vi "2021 Advent puzzle 02.vi"() -> ()   [LabVIEW 2021]
panel:
  out "output 1":string
  out "64bit integer":i64
  out "index 2":i64
  out "index":i64
  out "x*y":i64
  out "y":i64
  out "x":i64
  # "1451208"
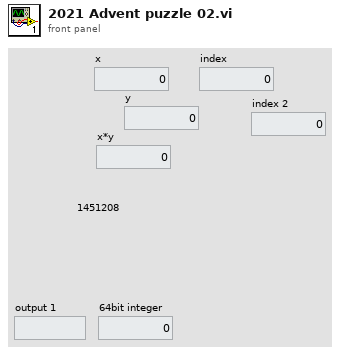
[diagram p1: front panel]
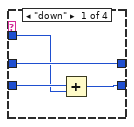
[diagram p2: hidden frame]
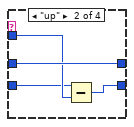
[diagram p3: hidden frame]
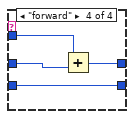
[diagram p4: hidden frame]
diagram:
  w5 = i64 0 ("index")
  (unwired) "forward 5\ndown 5\nforward 8\nup 3\ndown 8\nforward 2"
  # "find end position"
  n1 = Spreadsheet String To Array(delimiter (Tab)="\n", format string="", spreadsheet string="forward 9\ndown 3\ndown 8\nforward 2\nup 3\nforward 5\nup 8\ndown 2\ndown 5\nup 7\ndown 9\nforward 4\nup 5\ndown 9\nforward 2\nforward 2\nforward 8\ndown 6\nforward 2\nup 9\nup 5\ndown 2\nforward 5\ndown 8\nforward 3\nup 4\nforward 5\nforward 7\ndown 8\ndown 6\nup 7\ndown 3\nforward 4\nup 8\ndown 5\ndown 3\ndown 6\ndown 8\nforward 1\nforward 9\nforward 4\nup 7\ndown 4\nforward 7\nforward 3\nforward 9\ndown 1\ndown 3\nup 9\ndown 3\nforward 9\nup 6\nup 9\ndown 8\nup 3\ndown 1\nup 8\ndown 8\ndown 2\ndown 4\ndown 4\nup 3\ndown 6\ndown 1\ndown 3\nforward 1\nup 5\nforward 5\nforward 8\ndown 2\nforward 6\nforward 2\nup 7\nforward 6\ndown 8\nforward 6\nforward 5\nup 9\nforward 5\nup 5\nforward 9\ndown 2\ndown 4\ndown 3\ndown 8\nforward 9\nforward 6\nforward 2\nup 7\ndown 7\nup 3\nforward 4\nforward 5\ndown 7\nforward 5\nup 9\nforward 6\nforward 6\nforward 1\ndown 6\nforward 9\nup 2\ndown 7\ndown 8\ndown 6\nup 5\ndown 8\ndown 8\nforward 7\ndown 6\nup 5\ndown 9\ndown 3\nforward 2\ndown 4\nforward 8\ndown 5\nup 5\nforward 7\nup 2\nup 2\ndown 4\nforward 4\ndown 5\nup 8\ndown 2\nforward 4\ndown 9\nforward 8\ndown 5\ndown 6\ndown 7\nup 7\nup 5\nup 7\nforward 7\nforward 8\ndown 2\nforward 3\ndown 2\ndown 7\ndown 4\ndown 2\nforward 3\nforward 5\ndown 3\ndown 7\nup 7\ndown 7\nup 5\nforward 1\ndown 8\ndown 2\nup 4\nup 5\ndown 8\nforward 9\ndown 3\ndown 9\nforward 8\nforward 1\nforward 1\ndown 2\nup 9\ndown 2\nup 8\ndown 6\nup 8\nforward 7\ndown 5\nforward 7\ndown 8\nforward 8\ndown 7\nup 9\nup 2\nup 6\ndown 5\ndown 9\nforward 2\nup 3\ndown 4\nup 5\nup 4\ndown 9\nforward 7\nforward 7\ndown 3\nforward 4\nforward 9\nup 8\nforward 3\ndown 1\nforward 2\ndown 7\ndown 3\ndown 7\ndown 7\nforward 8\nforward 4\nforward 7\nup 1\ndown 4\nup 9\ndown 2\ndown 1\nforward 6\ndown 3\nforward 7\nforward 8\nup 9\nup 2\nup 2\nforward 7\nup 2\nup 5\nforward 5\ndown 3\nforward 8\nforward 1\nup 4\ndown 6\ndown 5\nforward 4\nup 9\nforward 8\nup 4\ndown 8\ndown 3\ndown 3\ndown 7\nforward 2\nforward 4\ndown 9\ndown 7\ndown 2\nup 3\nup 3\nforward 8\nforward 7\nforward 8\ndown 5\nup 5\nforward 3\nforward 6\nup 7\nup 1\nforward 2\nforward 5\ndown 5\nforward 8\ndown 2\ndown 4\nforward 2\ndown 7\ndown 3\ndown 5\nforward 9\ndown 7\ndown 8\nup 1\nup 2\ndown 8\nforward 7\nforward 8\ndown 8\nforward 5\nup 7\nforward 3\nup 2\ndown 7\nforward 1\ndown 2\nup 7\nup 4\ndown 2\nforward 1\nup 5\nforward 2\nup 2\nforward 3\nforward 9\nforward 2\nforward 8\nforward 2\nup 7\ndown 8\ndown 7\nforward 2\nforward 7\ndown 1\nforward 2\nup 1\nup 6\ndown 3\ndown 6\nforward 7\ndown 4\nforward 5\nforward 6\nup 3\nforward 3\ndown 6\nforward 8\nup 8\nforward 4\ndown 3\nforward 3\ndown 4\ndown 7\nforward 9\nforward 2\nup 2\nforward 8\ndown 6\nforward 6\ndown 9\ndown 9\nforward 8\ndown 1\nforward 9\ndown 1\ndown 6\ndown 8\ndown 5\ndown 5\nforward 3\nforward 3\ndown 2\ndown 5\nforward 9\ndown 2\ndown 8\ndown 3\nforward 9\nup 2\ndown 4\ndown 9\nforward 9\nforward 1\nforward 5\nup 9\ndown 1\ndown 6\nforward 6\nforward 5\nforward 8\ndown 2\nforward 8\ndown 4\ndown 2\ndown 6\ndown 6\nup 3\nup 8\nforward 1\ndown 1\nup 8\ndown 3\ndown 4\nup 9\nup 1\ndown 7\ndown 7\nup 1\nup 2\nforward 5\nup 8\nforward 2\ndown 3\nforward 1\nup 5\nforward 6\nforward 2\ndown 6\nup 2\nforward 2\nforward 1\ndown 3\nforward 4\nup 8\nforward 5\ndown 4\nforward 2\ndown 8\ndown 7\nup 7\ndown 8\nforward 1\ndown 4\nup 9\ndown 6\nup 6\nup 6\ndown 2\nforward 1\nforward 8\ndown 6\nup 3\ndown 7\nforward 9\nup 1\nup 4\nforward 7\ndown 7\nforward 1\ndown 6\ndown 4\ndown 7\ndown 8\ndown 8\nforward 4\ndown 6\ndown 6\ndown 5\nforward 6\nup 9\nup 3\ndown 4\nforward 8\ndown 7\nforward 6\nup 3\nforward 1\nforward 1\ndown 8\nforward 7\nforward 4\nforward 6\nup 1\nforward 7\nup 8\nforward 2\nforward 6\nforward 8\ndown 9\ndown 8\nup 9\nup 4\nup 2\nforward 2\nforward 8\nup 2\nforward 3\nforward 2\nup 2\nup 5\nup 8\nforward 4\nforward 8\nforward 3\nup 5\ndown 1\nforward 2\ndown 7\ndown 8\nforward 3\nup 1\nforward 5\nforward 7\nforward 9\nup 7\nforward 4\ndown 4\nup 2\nforward 4\nforward 5\nforward 3\nup 9\nforward 6\nforward 8\ndown 9\ndown 1\nforward 1\ndown 5\ndown 2\nforward 9\ndown 2\nup 9\ndown 1\nforward 5\nforward 8\nup 2\nforward 6\ndown 4\ndown 9\nforward 4\nforward 1\ndown 3\ndown 3\nup 5\nforward 5\ndown 6\nforward 3\ndown 2\nforward 8\ndown 7\ndown 2\ndown 1\nforward 2\nup 5\nforward 9\nforward 3\nforward 5\ndown 4\nup 7\nforward 6\ndown 3\nforward 1\nforward 7\nforward 1\nup 4\ndown 2\ndown 7\nup 9\nforward 9\ndown 8\ndown 1\nup 2\ndown 3\nforward 7\ndown 8\ndown 5\ndown 5\nup 8\nforward 1\ndown 5\nforward 8\nup 7\ndown 1\nforward 9\ndown 4\nforward 8\nforward 5\nforward 7\nforward 8\nforward 3\nup 9\nforward 3\ndown 7\ndown 5\nup 8\nforward 3\nup 6\nforward 8\nup 3\ndown 5\nforward 5\nforward 6\nforward 4\nforward 3\nforward 8\nup 9\nforward 2\ndown 6\ndown 4\ndown 5\nforward 7\ndown 2\nup 5\nforward 2\nforward 5\ndown 9\nforward 8\ndown 8\nforward 6\ndown 9\ndown 7\nup 9\nforward 3\nforward 3\nup 5\ndown 2\nforward 5\ndown 6\ndown 6\ndown 2\ndown 3\ndown 4\nforward 7\nup 1\ndown 7\nforward 7\nup 1\nforward 3\nup 6\ndown 7\ndown 5\nforward 9\nforward 2\ndown 5\nforward 9\ndown 5\nforward 9\nforward 1\ndown 4\nforward 9\ndown 5\nforward 8\ndown 6\ndown 4\ndown 5\nforward 9\ndown 1\nforward 6\nforward 9\ndown 1\ndown 1\nup 2\nforward 5\nforward 3\ndown 4\nup 8\nforward 8\ndown 2\nforward 3\nforward 1\ndown 7\nforward 6\nforward 5\nup 7\nup 8\ndown 5\nup 3\ndown 8\nforward 6\nforward 5\nforward 6\nup 1\nup 8\nup 7\ndown 5\nforward 3\nforward 9\nup 9\nup 4\nup 7\nup 8\nforward 7\nforward 3\nforward 9\ndown 7\nforward 3\ndown 6\nforward 9\ndown 1\nforward 3\ndown 1\nforward 8\nforward 7\ndown 2\nforward 1\nforward 6\nforward 7\ndown 3\ndown 2\ndown 1\nforward 7\nforward 4\ndown 6\nup 4\nforward 4\nforward 9\nforward 3\ndown 1\nup 2\ndown 3\ndown 5\nforward 7\nforward 5\nup 1\ndown 2\ndown 3\ndown 8\nforward 1\ndown 4\nforward 5\ndown 5\nup 6\ndown 6\ndown 8\nforward 1\nforward 9\nup 5\nforward 2\ndown 9\ndown 5\ndown 1\ndown 4\ndown 9\ndown 8\nforward 2\nforward 4\nup 2\nforward 3\ndown 8\ndown 5\nup 5\nforward 8\nup 2\ndown 8\nup 3\nforward 7\ndown 7\nforward 8\ndown 7\ndown 3\nup 6\nforward 5\nup 4\nup 5\nforward 9\nforward 6\ndown 9\nforward 5\ndown 5\ndown 3\nforward 2\ndown 1\nup 9\nup 8\ndown 6\ndown 1\nforward 9\nforward 4\nforward 2\nup 1\nforward 5\nforward 9\nup 5\nforward 8\nforward 4\ndown 4\ndown 4\ndown 2\nforward 1\nforward 7\ndown 9\nforward 4\ndown 5\ndown 4\ndown 7\ndown 2\nforward 9\ndown 3\nforward 6\nforward 3\ndown 9\ndown 3\ndown 4\ndown 9\ndown 9\nup 6\ndown 5\nup 4\ndown 1\ndown 1\nforward 9\nforward 7\ndown 9\nforward 4\ndown 8\ndown 7\nforward 7\nforward 4\nup 2\nup 5\nforward 2\nforward 7\ndown 1\nforward 6\nforward 6\nforward 3\nforward 8\ndown 2\nup 2\nforward 7\nup 5\ndown 1\ndown 5\nforward 8\ndown 6\nforward 8\ndown 5\ndown 4\ndown 6\nforward 5\ndown 1\nforward 9\nforward 8\nup 5\ndown 6\nforward 5\nup 5\ndown 4\nforward 1\ndown 2\ndown 5\ndown 3\nforward 2\ndown 9\nforward 1\nforward 1\nforward 1\nforward 8\nforward 2\ndown 8\ndown 6\nup 1\nforward 6\ndown 3\ndown 4\nup 9\ndown 3\ndown 3\nup 7\ndown 4\nforward 4\nforward 9\ndown 3\ndown 8\nforward 5\ndown 3\ndown 6\ndown 7\nforward 1\nup 2\nforward 8\ndown 1\ndown 4\nup 9\nforward 9\nup 4\nup 2\nforward 3\nforward 4\ndown 2\ndown 2\ndown 6\nforward 6\nforward 8\ndown 6\nup 6\ndown 5\nforward 1\ndown 4\nup 9\nforward 1\nforward 3\ndown 1\ndown 4\nup 6\nforward 5\nforward 6\nup 9\nup 9\ndown 2\nup 6\nforward 1\nforward 2\nforward 3\nforward 3\nforward 6\nup 2\ndown 8\ndown 9\nforward 7\nup 1\nup 3\ndown 2\nforward 3\ndown 8\nforward 9\ndown 3\nforward 6\nup 2\nforward 7\ndown 2\nforward 5\ndown 4\ndown 2\nup 8\nforward 3\nforward 5\nforward 9\nforward 5\nforward 3\nup 9\ndown 7\nforward 4\nforward 2\nforward 7\ndown 5\nup 6\nup 6\nforward 8\ndown 2\nforward 1\nup 1\nup 9\nup 8\nup 3\nup 4\ndown 2\nup 7\ndown 4\nup 5\ndown 1\nup 9\ndown 5\ndown 9\ndown 4\nup 2\ndown 8\nup 2\nup 7\nup 9\nforward 4\nforward 2\nforward 1\nforward 6\nforward 8\nup 5\nforward 5\nforward 5\ndown 4\nup 6\nforward 3\ndown 9\ndown 7\nforward 4\ndown 3\nup 1\nforward 4\ndown 2\ndown 6\nup 3\nup 1\ndown 9\ndown 7\ndown 9\nforward 3\nforward 8\ndown 8\nup 7\nup 6\ndown 2\ndown 9\ndown 1\ndown 9\nforward 6\nup 4\ndown 3\nforward 5\nup 3\nup 9\nup 8\nforward 6\ndown 8\nforward 6\nforward 6\nforward 5\nup 4\ndown 4\nup 6\nup 4\nforward 2\ndown 5\nforward 9\nup 7\nup 6\ndown 4\nforward 7\nforward 6\nup 2\ndown 8\ndown 6\nforward 5\nup 2\nforward 5\nforward 1\nup 9\ndown 8\nforward 7\nup 4\nforward 8\ndown 4\nforward 3\nforward 3\ndown 9\nforward 4\nforward 9\nup 8\nforward 7\nforward 3\nforward 9\nforward 4\nup 3\nforward 2\nforward 7", array type (2D Dbl)=string[] []) -> (array=w6:string[])
  n2 = for {
    tunnel: w6 -> [w19] mode=indexing
    shift-right: [w13] -> w4
    shift-left: w5 -> [w15]
    shift-right: [w12] -> w3
    shift-left: w5 -> [w14]
    tunnel: [w10] -> _ mode=indexing
    i -> [w10]
    # "y"
    # "x"
    n3 = Scan From String(format string="%s %d", input string=w19) -> (output 1=w17:string, output 2=w16:i32)  [unwired: 4 in, 3 out]
    "output 1" <- w17
    n4 = To Quad Integer(1:w16) -> (0:w11:i64)
    "64bit integer" <- w11
    n5 = case shown="Default" w17 {
      tunnel: w11 -> [w20 w26 _ w30]
      tunnel: w15 -> [w23 w27 w29 w33]
      tunnel: w14 -> [w22 w24 w28 w32]
      tunnel: [w23 w27 w29 w31] -> w13
      tunnel: [w21 w25 w28 w32] -> w12
      frame "down" {
        n6 = Add(x=w22, y=w20) -> (x+y=w21:i64)
      }
      frame "up" {
        n7 = Subtract(x=w24, y=w26) -> (x-y=w25:i64)
      }
      frame Default {
      }
      frame "forward" {
        n8 = Add(x=w30, y=w33) -> (x+y=w31:i64)
      }
    }
    "index" <- w12
    "index 2" <- w13
  }
  "x" <- w4
  "y" <- w3
  n9 = Multiply(x=w4, y=w3) -> (x*y=→"x*y":i64)
